vi "Delete All Children.vi"(8 "error in (no error)":errorcluster, 11 "Item Ref in":T1 format="%.0x") -> (0 "error out":errorcluster, 3 "Item Ref out":T1 format="%.0x")   [LabVIEW 2019, in "DSF System Explorer.lvlib"]
uses:
  DSF System Explorer.lvlib
  <vilib>/NI VeriStand/Custom Device API/Custom Device Item Ref.ctl
  <vilib>/NI VeriStand/Custom Device API/Custom Device API.lvlib
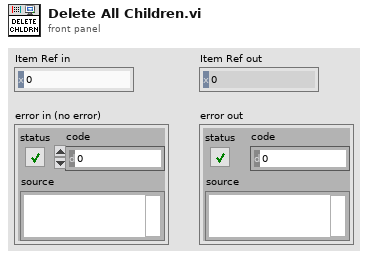
[diagram p1: front panel]
types:
  T1 = typedef "Custom Device API.lvlib/Custom Device Item Ref.ctl" = u64
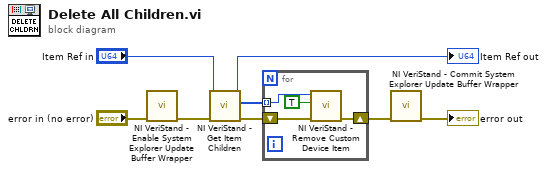
[diagram p0: block diagram]
diagram:
  n1 = call "NI VeriStand - Enable System Explorer Update Buffer Wrapper.vi"("error in"="error in (no error)") -> ("error out"=w1:errorcluster)  [unwired: 10 in]
  n2 = call <vilib>:"NI VeriStand - Get Item Children.vi"("error in (no error)"=w1, "Item Ref in"="Item Ref in") -> ("error out"=w5:errorcluster, "Child Refs"=w6:T1[], "Item Ref out"=→"Item Ref out":T1)  [unwired: 6 in, 1 out]
  n3 = for {
    tunnel: w6 -> [w11] mode=indexing
    shift-right: [w10] -> w4
    shift-left: w5 -> [w12]
    n4 = call <vilib>:"NI VeriStand - Remove Custom Device Item.vi"("error in (no error)"=w12, "Force Delete (F)"=TRUE, "Item Ref in"=w11) -> ("error out"=w10:errorcluster)  [unwired: 7 in, 1 out]
  }
  n5 = call "NI VeriStand - Commit System Explorer Update Buffer Wrapper.vi"("error in"=w4) -> ("error out"=→"error out":errorcluster)  [unwired: 10 in]
